vi "Q_Delete.vi"(8 "error in":errorcluster caption="错误输入（无错误）", 10 "CloseVI?(T)":bool=TRUE, 11 "ChildNode*":refnum<data-value>) -> (0 "error out":errorcluster caption="错误输出")   [LabVIEW 2016, in "PanelDataNode.lvclass"]
uses:
  PanelDataNode.lvclass
  PanelDataNode.lvclass/PanelDataNode.ctl
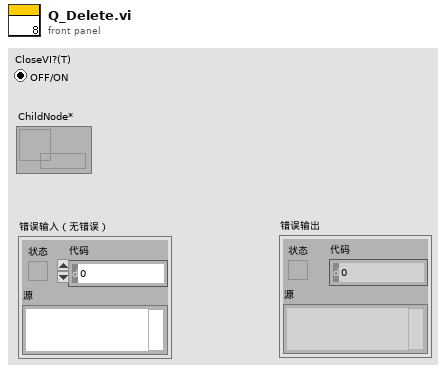
[diagram p1: front panel]
types:
  T1 = cluster{"ChildNode*":refnum<data-value>, "CloseVI?(T)":bool}
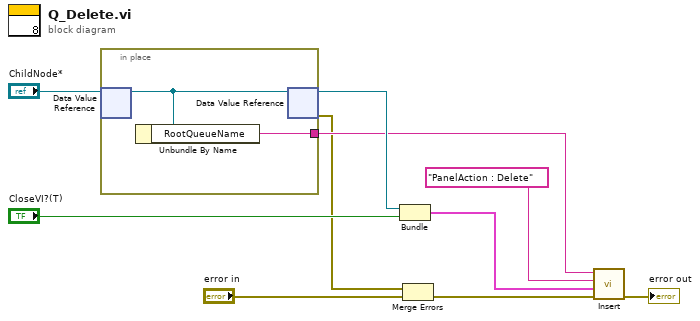
[diagram p0: block diagram]
diagram:
  n1 = in-place {
    in-place-border: [w11] -> w6
    n2 = in-place-dvr #1("ChildNode*") -> (w12:refnum<class "PanelDataNode.lvclass">)  [unwired: 1 out]
    n3 = Unbundle By Name(w12) -> ("RootQueueName"=w11:string)
    n4 = in-place-dvr #1(w12) -> (w7:refnum<data-value>, w1:errorcluster)
  }
  n5 = Bundle("ChildNode*"=w7, "CloseVI?(T)"="CloseVI?(T)") -> (w10:T1)  [unwired: 1 in]
  n6 = Merge Errors(w1, "error in") -> (w2:errorcluster)
  n7 = call "Insert.vi"("error in"=w2, "Data"=w10, "Event"="PanelAction : Delete", "QueueName"=w6) -> ("error out"=→"error out":errorcluster)  [unwired: 6 in, 1 out]
